vi "led_on.vi"(8 "CurrentState":string, 11 "Action":enum16{"Entry", "During", "Exit"}(ring)) -> (0 "NextState":string)   [LabVIEW 2021]
uses:
  led_globals.vi
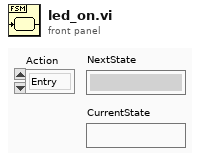
[diagram p1: front panel]
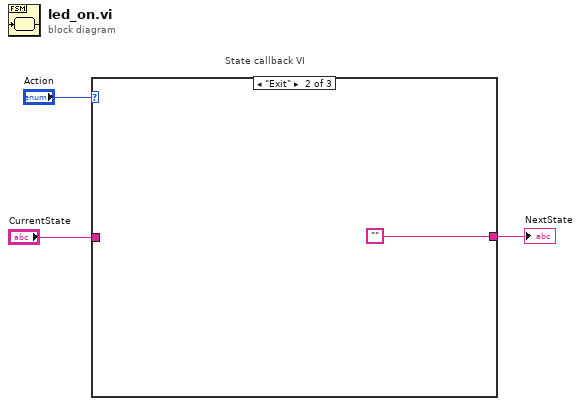
[diagram p0: block diagram]
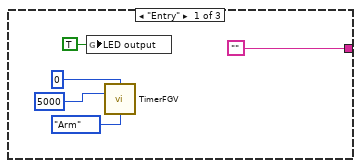
[diagram p2: hidden frame]
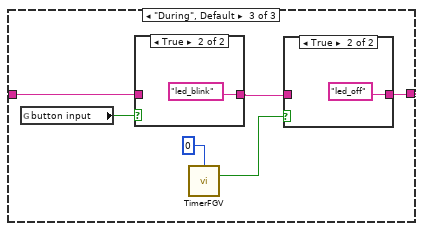
[diagram p3: hidden frame]
diagram:
  # "State callback VI"
  n1 = case shown="\"Exit\"" "Action" {
    tunnel: ["" "" w12] -> w2
    tunnel: "CurrentState" -> [_ _ w14]
    frame "Entry" {
      n2 = global write "led_globals.vi" "LED output"(TRUE ("LED output")) -> ()
      n3 = call "TimerFGV.vi"("index"=0, "time(ms)"=u32 5000, "action"=enum16{"Check", "Arm", "Disarm", "Init"}."Arm") -> ()  [unwired: 10 in, 3 out]
    }
    frame "Exit" {
    }
    frame "During", Default {
      n4 = global read "led_globals.vi" "button input"() -> (w15:bool)
      n5 = case shown="True" w15 {
        tunnel: [w18 "led_blink"] -> w13
        tunnel: w14 -> [w18 _]
        frame False {
        }
        frame True {
        }
      }
      n6 = call "TimerFGV.vi"("index"=0) -> ("expired?"=w11:bool)  [unwired: 12 in, 2 out]
      n7 = case shown="True" w11 {
        tunnel: [w16 "led_off"] -> w12
        tunnel: w13 -> [w16 _]
        frame False {
        }
        frame True {
        }
      }
    }
  }
  "NextState" <- w2
